vi "TEMOCR-Close IPC.vi"(7 "IPC":T1) -> ()   [LabVIEW 2015]
uses:
  Typedefs/TEMOCR-IPC.ctl
  Typedefs/TEMOCR-Parameters.ctl
  Typedefs/TEMOCR-Probe.ctl
  Typedefs/TEMOCR-Elicitor.ctl
  Human Studies/SFM Frontend/LV Source/Typedefs/HSTS-Transducer.ctl
  Typedefs/TEMOCR-Sequence.ctl
  Typedefs/TEMOCR-Analysis.ctl
  CFTS Main Panel SubVIs/CFTS-Experiment State.ctl
  Typedefs/TEMOCR-Sequence Step.ctl
panel:
  out "error out":errorcluster
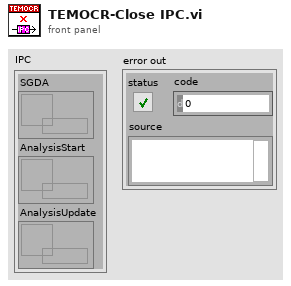
[diagram p1: front panel]
types:
  T1 = typedef "TEMOCR-IPC.ctl" = cluster{"SGDA":refnum<queue>, "AnalysisStart":refnum<queue>, "AnalysisUpdate":refnum<queue>}
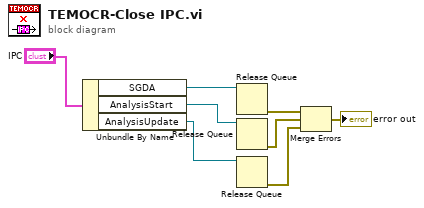
[diagram p0: block diagram]
diagram:
  n1 = Unbundle By Name("IPC") -> ("SGDA"=w7:refnum<queue>, "AnalysisStart"=w6:refnum<queue>, "AnalysisUpdate"=w5:refnum<queue>)
  n2 = Release Queue(queue=w7) -> (error out=w4:errorcluster)  [unwired: 2 in, 2 out]
  n3 = Release Queue(queue=w6) -> (error out=w3:errorcluster)  [unwired: 2 in, 2 out]
  n4 = Release Queue(queue=w5) -> (error out=w2:errorcluster)  [unwired: 2 in, 2 out]
  n5 = Merge Errors(w4, w3, w2) -> (→"error out":errorcluster)
